vi "Generate Report.vi"(8 "error in (no error)":errorcluster, 11 "XML Report In":refnum<class "XML Report.lvclass">) -> (0 "error out":errorcluster, 3 "XML Report Out":refnum<class "XML Report.lvclass">)   [LabVIEW 2020, in "Reports.lvlib" / "XML Report.lvclass"]
uses:
  XML Report.lvclass
  XML Report.lvclass/XML Report.ctl
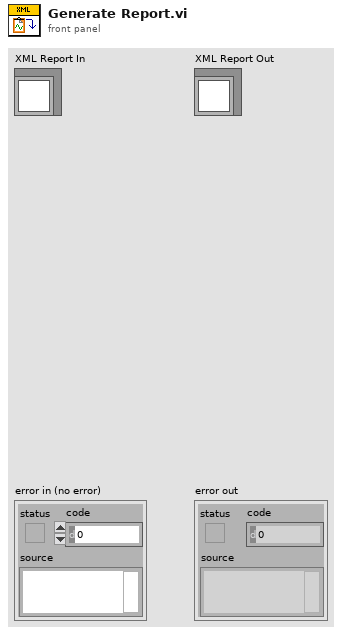
[diagram p1: front panel]
types:
  T1 = typedef "Reports.lvlib/XML Report.lvclass/Case Result.ctl" = cluster{"Name":string, "Assertions":i32, "Classname":string, "Status":T2, "Time":dbl}
  T2 = typedef "Result.lvlib/Status.ctl" = enum16{"", "Passed", "Failed", "Error", "Skipped", "Setup Error", "Broken", "Teardown Error"}
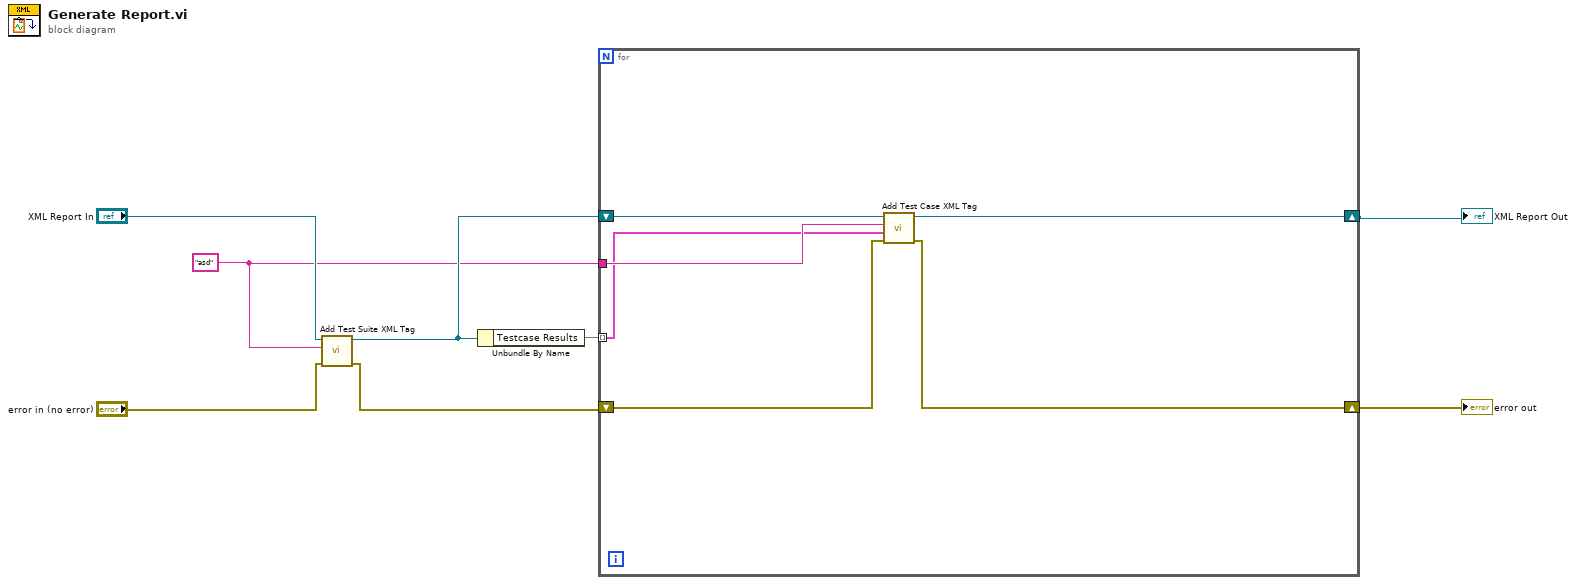
[diagram p0: block diagram]
diagram:
  w1 = "asd" ("Tag Name")
  n1 = call "Add Test Suite XML Tag.vi"("error in (no error)"="error in (no error)", "Suite Name"=w1, "Reports.lvlib:XML Report.lvclass"="XML Report In") -> ("error out"=w5:errorcluster, "output cluster"=w7:refnum<class "XML Report.lvclass">)  [unwired: 7 in]
  n2 = Unbundle By Name(w7) -> ("Testcase Results"=w2:map{string, T1})
  n3 = for {
    shift-right: [w11] -> w3
    shift-left: w5 -> [w12]
    shift-right: [w13] -> w4
    shift-left: w7 -> [w14]
    tunnel: w2 -> [w9] mode=indexing
    tunnel: w1 -> [w10]
    n4 = call "Add Test Case XML Tag.vi"("error in (no error)"=w12, "Test Case Result"=w9, "Owning Suite"=w10, "Reports.lvlib:XML Report.lvclass"=w14) -> ("error out"=w11:errorcluster, "output cluster"=w13:refnum<class "XML Report.lvclass">)  [unwired: 6 in]
  }
  "error out" <- w3
  "XML Report Out" <- w4
